vi "GetArrayType.vi"(8 "error in (no error)":errorcluster, 11 "Control in":refnum<vi>) -> (0 "error out":errorcluster, 2 "Type":string, 3 "Control out":refnum<vi>)   [LabVIEW 2019]
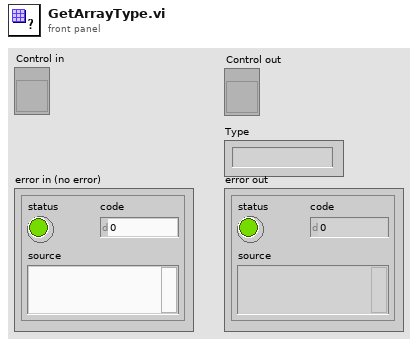
[diagram p1: front panel]
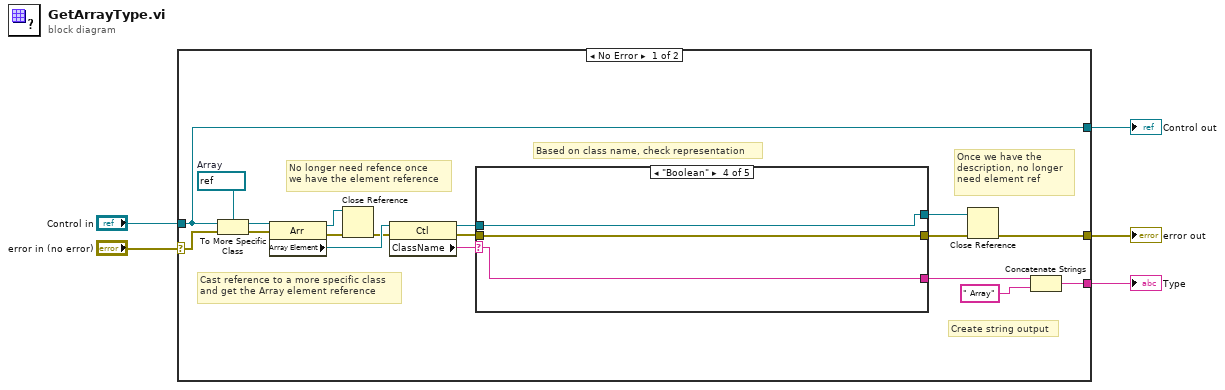
[diagram p0: block diagram]
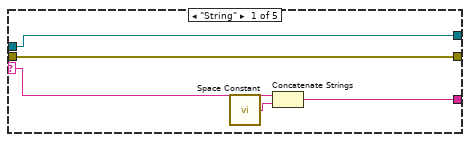
[diagram p2: hidden frame]
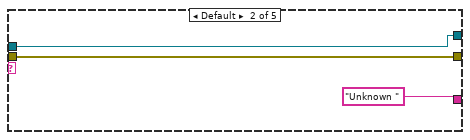
[diagram p3: hidden frame]
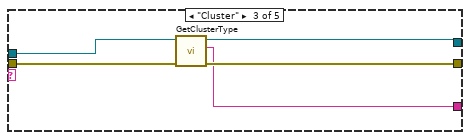
[diagram p4: hidden frame]
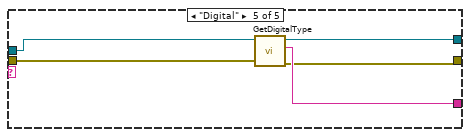
[diagram p5: hidden frame]
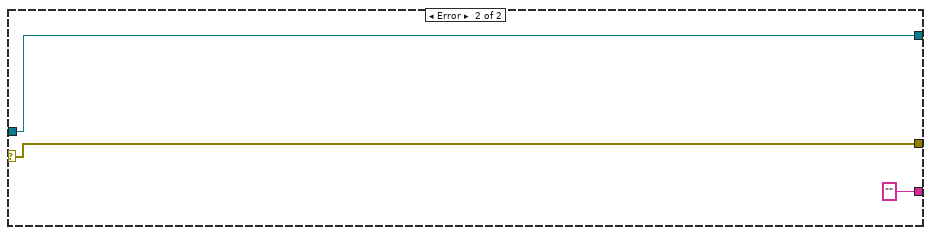
[diagram p6: hidden frame]
diagram:
  n1 = case shown="No Error" "error in (no error)" {
    selector: "error in (no error)" -> [w13 w47]
    tunnel: "Control in" -> [w12 w45]
    tunnel: [w12 w45] -> w1
    tunnel: [w6 w47] -> w4
    tunnel: [w14 ""] -> w3
    frame No Error {
      w18 = refnum<vi> refnum  # Array
      # "Create string output"
      # "Once we have the \ndescription, no longer\nneed element ref"
      # "Based on class name, check representation"
      # "Cast reference to a more specific class\nand get the Array element reference"
      # "No longer need refence once \nwe have the element reference"
      n2 = To More Specific Class(target class=w18, reference=w12, error in=w13) -> (specific class reference=w19:refnum<vi>, error out=w20:errorcluster)
      n3 = property class="Arr"(reference=w19, error in=w20) -> (reference out=w11:refnum<vi>, error out=w10:errorcluster, "Array Element"=w21:refnum<vi>)
      n4 = Close Reference(reference=w11, error in (no error)=w10) -> (error out=w9:errorcluster)
      n5 = property class="Ctl"(reference=w21, error in=w9) -> (reference out=w23:refnum<vi>, error out=w17:errorcluster, "ClassName"=w22:string)
      n6 = case shown="\"Boolean\"" w22 {
        selector: w22 -> [w28 _ _ w39 _]
        tunnel: [w27 "Unknown " w32 w39 w44] -> w16
        tunnel: w23 -> [w24 w29 w36 w37 w43]
        tunnel: w17 -> [w25 w30 w35 w38 w42]
        tunnel: [w25 w30 w34 w38 w41] -> w7
        tunnel: [w24 w29 w33 w37 w40] -> w8
        frame "String" {
          n7 = call <vilib>:"Space Constant.vi"() -> ("String"=w26:string)
          n8 = Concatenate Strings(w28, w26) -> (w27:string)
        }
        frame Default {
        }
        frame "Cluster" {
          n9 = call "GetClusterType.vi"("error in"=w35, "Control in"=w36) -> ("error out"=w34:errorcluster, "Cluster Type"=w32:string, "Control out"=w33:refnum<vi>)  [unwired: 7 in]
        }
        frame "Boolean" {
        }
        frame "Digital" {
          n10 = call "GetDigitalType.vi"("error in (no error)"=w42, "Control in"=w43) -> ("error out"=w41:errorcluster, "String"=w44:string, "Control in 2"=w40:refnum<vi>)  [unwired: 7 in]
        }
      }
      n11 = Close Reference(reference=w8, error in (no error)=w7) -> (error out=w6:errorcluster)
      n12 = Concatenate Strings(w16, " Array" ("string")) -> (w14:string)
    }
    frame Error {
    }
  }
  "Type" <- w3
  "error out" <- w4
  "Control out" <- w1
